vi "Wait Until Act.vi"(0 "Data Acq":T1=enum."NML Data Acquisition-New.vi", 1 "command text in":string[](array[string])) -> ()   [LabVIEW 2025]
doc: "Author: Scott Hannahs <sth@magnet.fsu.edu>\n\nThis software is licensed for use under the “MIT License\"\nCopyright (c) 2025 Scott Hannahs, sth@sth@magnet.sthnet.net\n\nPermission is hereby granted, free of charge, to any person obtaining a copy of this software and associated documentation files (the \"Software\"), to deal in the Software without restriction, including without limitation the rights to use, copy, modify, merge, publish, distribute, sublicense, and/or sell copies of the Software, and to permit persons to whom the Software is furnished to do so, subject to the following conditions: The above copyright notice and this permission notice shall be included in all copies or substantial portions of the Software.\n\nTHE SOFTWARE IS PROVIDED \"AS IS\", WITHOUT WARRANTY OF ANY KIND, EXPRESS OR IMPLIED, INCLUDING BUT NOT LIMITED TO THE WARRANTIES OF MERCHANTABILITY, FITNESS FOR A PARTICULAR PURPOSE AND NONINFRINGEMENT. IN NO EVENT SHALL THE AUTHORS OR COPYRIGHT HOLDERS BE LIABLE FOR ANY CLAIM, DAMAGES OR OTHER LIABILITY, WHETHER IN AN ACTION OF CONTRACT, TORT OR OTHERWISE, ARISING FROM, OUT OF OR IN CONNECTION WITH THE SOFTWARE OR THE USE OR OTHER DEALINGS IN THE SOFTWARE."
uses:
  Ctl/Data Acquisition System.ctl
panel:
  out "initial value":dbl
  out "monitorng value":dbl
  in  "update every (s)":dbl=0.5
  out "Timeout (sec)":dbl=10000.0
  out "Target Value":dbl
  out "xxx%":dbl
  out "index":i32
  out "Condition":T2(ring)=enum."= target value"
  out "data":dbl[](array[numeric])
  out "error out":errorcluster
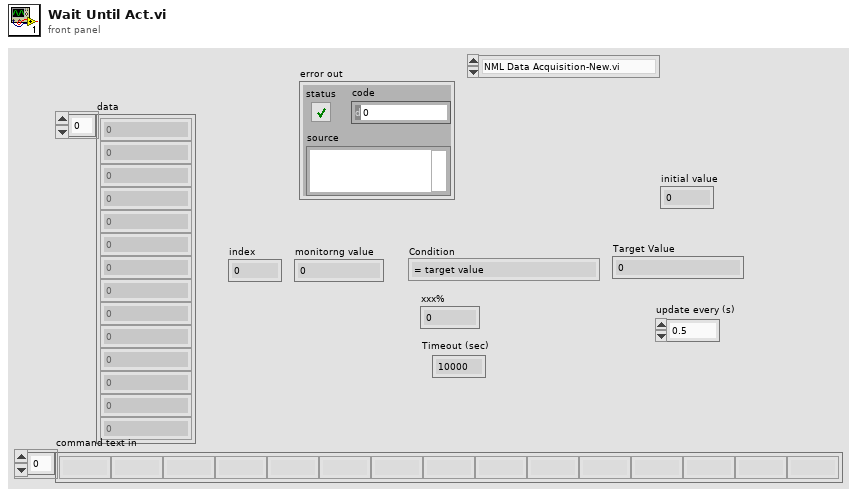
[diagram p1: front panel]
types:
  T1 = typedef "Data Acquisition System.ctl" = enum16{"NML Data Acquisition-old.vi", "NML Data Acquisition-New.vi"}
  T2 = enum16{"within xxx% of target value", "<= target value", ">= target value", "= target value"}
  T3 = typedef "Wait Until.ctl" = cluster{"Available Data":string[], "Target Value":dbl, "Condition":T4, "xxx%":dbl, "Timeout (sec)":dbl, "selected index":u32, "initial wait (sec)":dbl}
  T4 = typedef "Wait Until condition.ctl" = enum16{"within xxx% of target value", "<= target value", ">= target value", "= target value"}
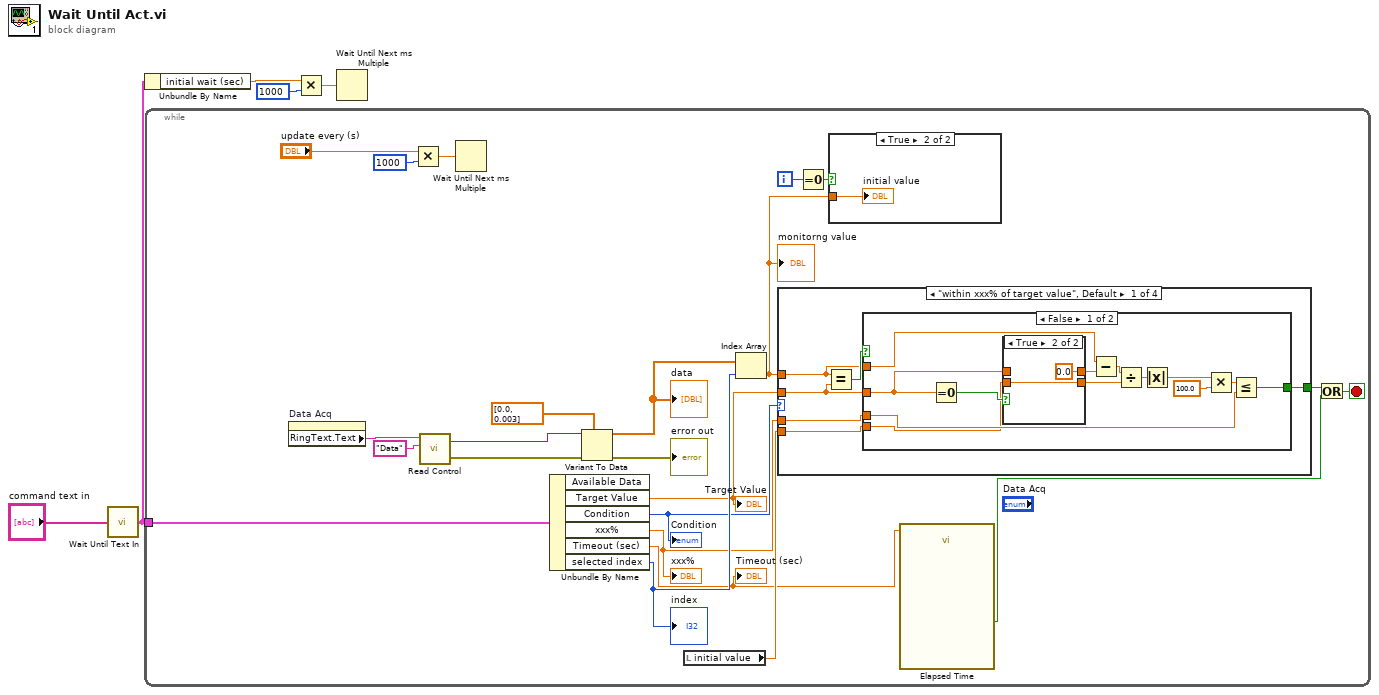
[diagram p0: block diagram]
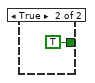
[diagram p4: hidden frame]
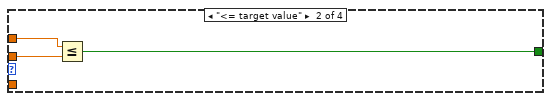
[diagram p5: hidden frame]
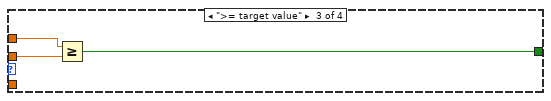
[diagram p6: hidden frame]
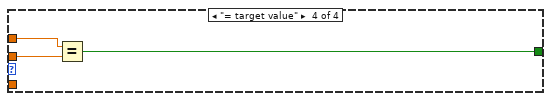
[diagram p7: hidden frame]
diagram:
  n1 = call "Wait Until Text In.vi"("command text in"="command text in") -> ("Wait Until Ctr"=w4:T3)
  n2 = Unbundle By Name(w4) -> ("initial wait (sec)"=w1:dbl)
  n3 = while {
    tunnel: w4 -> [w11]
    i -> [w16]
    stop <- w12 stop-if-true
    n4 = property on="Data Acq" class="Enum (strict)"() -> ("RingText.Text"=w13:string)  [unwired: 2 in, 2 out]
    n5 = Multiply(x="update every (s)", y=1000) -> (x*y=w22:dbl)
    n6 = call "Read Control.vi"("VI Name"=w13, "Control Name"="Data") -> ("Value"=w28:variant, "error out"=w27:errorcluster)  [unwired: 3 in]
    n7 = Wait Until Next ms Multiple(millisecond multiple=w22) -> ()  [unwired: 1 out]
    n8 = Unbundle By Name(w11) -> ("Target Value"=w8:dbl, "Condition"=w9:T4, "xxx%"=w7:dbl, "Timeout (sec)"=w6:dbl, "selected index"=w10:u32)  [unwired: 1 out]
    "Condition" <- w9
    "index" <- w10
    "xxx%" <- w7
    "Target Value" <- w8
    "Timeout (sec)" <- w6
    n9 = Variant To Data(error in=w27, type=dbl[] [0.0, 0.003] ("Data"), Variant=w28) -> (data=w24:dbl[], error out=→"error out":errorcluster)
    "data" <- w24
    n10 = local read "initial value"() -> (w14:dbl)
    n11 = Index Array(array=w24, index=w10) -> (element=w15:dbl)
    "monitorng value" <- w15
    n12 = case shown="\"within xxx% of target value\", Default" w9 {
      tunnel: w8 -> [w33 w53 w56 w59]
      tunnel: [w34 w55 w58 w61] -> w20
      tunnel: w7 -> [w32 _ _ _]
      tunnel: w15 -> [w31 w54 w57 w60]
      tunnel: w14 -> [w30 _ _ _]
      frame "within xxx% of target value", Default {
        n13 = Equal?(x=w31, y=w33) -> (x = y?=w35:bool)
        n14 = case shown="False" w35 {
          tunnel: [w40 TRUE] -> w34
          tunnel: w33 -> [w43 _]
          tunnel: w32 -> [w44 _]
          tunnel: w31 -> [w37 _]
          tunnel: w30 -> [w36 _]
          frame False {
            n15 = Equal To 0?(x=w43) -> (x = 0?=w48:bool)
            n16 = case shown="True" w48 {
              tunnel: [w49 0.0 ("Target Value")] -> w39
              tunnel: w43 -> [w49 _]
              tunnel: [w49 w50] -> w38
              tunnel: w36 -> [_ w50]
              frame False {
              }
              frame True {
              }
            }
            n17 = Subtract(x=w37, y=w39) -> (x-y=w41:dbl)
            n18 = Divide(x=w41, y=w38) -> (x/y=w42:dbl)
            n19 = Absolute Value(x=w42) -> (abs(x)=w45:dbl)
            n20 = Multiply(x=w45, y=100.0) -> (x*y=w46:dbl)
            n21 = Less Or Equal?(x=w46, y=w44) -> (x <= y?=w40:bool)
          }
          frame True {
          }
        }
      }
      frame "<= target value" {
        n22 = Less Or Equal?(x=w54, y=w53) -> (x <= y?=w55:bool)
      }
      frame ">= target value" {
        n23 = Greater Or Equal?(x=w57, y=w56) -> (x >= y?=w58:bool)
      }
      frame "= target value" {
        n24 = Equal?(x=w60, y=w59) -> (x = y?=w61:bool)
      }
    }
    n25 = Equal To 0?(x=w16) -> (x = 0?=w17:bool)
    n26 = case shown="True" w17 {
      tunnel: w15 -> [_ w29]
      frame False {
      }
      frame True {
        "initial value" <- w29
      }
    }
    n27 = call "Elapsed Time"("Time Target (s)"=w6) -> ("Time has Elapsed"=w19:bool)  [unwired: 11 in, 7 out]
    n28 = Or(x=w20, y=w19) -> (x .or. y?=w12:bool)
  }
  n29 = Multiply(x=w1, y=1000) -> (x*y=w2:dbl)
  n30 = Wait Until Next ms Multiple(millisecond multiple=w2) -> ()  [unwired: 1 out]
